vi "RetrieveMAXExample.vi"() -> ()   [LabVIEW 2017]
uses:
  <vilib>/addons/database/Connection.llb/DB Tools Open Connec (Path).vi
  <vilib>/addons/database/Connection.llb/Conn Execute.vi
  <vilib>/addons/database/Recordset.llb/Rec Fetch Recordset Data (R).vi
  <vilib>/addons/database/Recordset.llb/Rec Destroy - Connection.vi
  <vilib>/addons/database/_DB Variant To Data/Database Variant To Data.xnode
  <vilib>/addons/database/NI_Database_API.lvlib
panel:
  out "element":dbl
  out "Variant data":variant[][](array[variant])
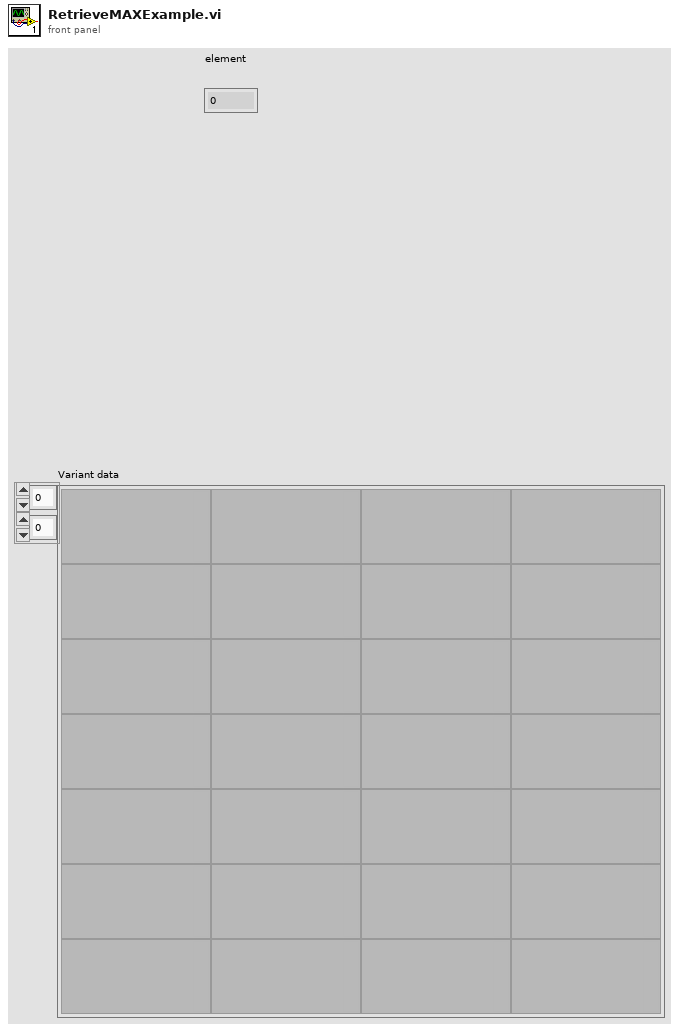
[diagram p1: front panel]
types:
  T1 = typedef "NI_Database_API.lvlib/Conn ObjectReference.ctl" = refnum<k1>
  T2 = typedef "NI_Database_API.lvlib/Rec ObjectReference.ctl" = refnum<k1>
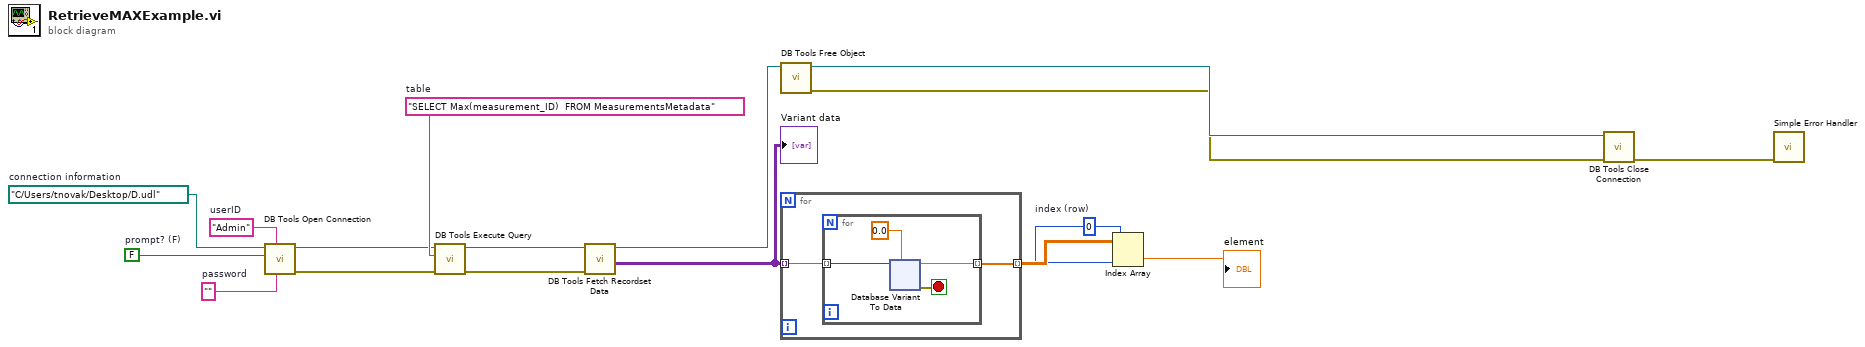
[diagram p0: block diagram]
diagram:
  w2 = 0  # index (row)
  w13 = path "C:/Users/tnovak/Desktop/D.udl"  # connection information
  w10 = ""  # password
  w12 = FALSE  # prompt? (F)
  w11 = "Admin"  # userID
  w14 = "SELECT Max(measurement_ID)  FROM MeasurementsMetadata"  # table
  n1 = call-poly <vilib>:"DB Tools Open Connection.vi"("password"=w10, "userID"=w11, "prompt? (F)"=w12, "connection information"=w13) -> ("error out"=w7:errorcluster, "connection reference"=w8:T1)  [unwired: 4 in]
  n2 = call-poly <vilib>:"DB Tools Execute Query.vi"("error in (no error)"=w7, "SQL query"=w14, "connection reference"=w8) -> ("error out"=w6:errorcluster, "recordset reference"=w15:T2)  [unwired: 5 in]
  n3 = call-poly <vilib>:"DB Tools Fetch Recordset Data.vi"("error in (no error)"=w6, "recordset reference"=w15) -> ("recordset data"=w17:variant[][], "recordset reference out"=w16:T2)  [unwired: 3 in, 1 out]
  "Variant data" <- w17
  n4 = call-poly <vilib>:"DB Tools Free Object.vi"("recordset reference"=w16) -> ("error out"=w4:errorcluster, "connection reference"=w5:T1)  [unwired: 9 in]
  n5 = for {
    tunnel: w17 -> [w19] mode=indexing
    tunnel: [w18] -> w3 mode=indexing
    n6 = for {
      tunnel: w19 -> [w23] mode=indexing
      tunnel: [w22] -> w18 mode=indexing
      stop <- w21 stop-if-true
      n7 = xnode "Database Variant To Data"("database variant"=w23, "type"=0.0) -> ("data"=w22:dbl, "error out"=w21:errorcluster)  [unwired: 1 in]
    }
  }
  n8 = Index Array(array=w3, index (row)=w2, index (col)=w2) -> (element=→"element":dbl)
  n9 = call <vilib>:"DB Tools Close Connection.vi"("error in (no error)"=w4, "connection reference"=w5) -> ("error out"=w9:errorcluster)  [unwired: 5 in]
  n10 = call <vilib>:"Simple Error Handler.vi"("error in (no error)"=w9) -> ()  [unwired: 4 in, 5 out]
